vi "Run Test Method.vi"(8 "error in (no error)":errorcluster, 11 "LUnit Test Case In":refnum<class "LUnit Inheriting Test Case.lvclass">) -> (0 "error out":errorcluster, 1 "Execution Time":dbl, 3 "LUnit Test Case Out":refnum<class "LUnit Inheriting Test Case.lvclass">)   [LabVIEW 2020]
uses:
  LUnit Inheriting Test Case.lvclass
  C:/git/astemes-lunit/source/API/LUnit Test Case/LUnit Test Case.lvclass
  C:/git/astemes-lunit/source/Core/Runnable/Runnable.lvclass
  C:/git/astemes-lunit/source/API/LUnit Inheriting Test Case/LUnit Test Case/LUnit Inheriting Test Case.lvclass
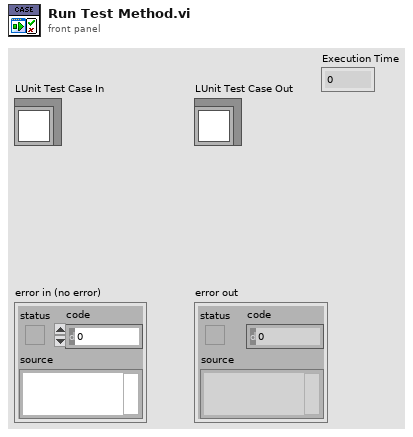
[diagram p1: front panel]
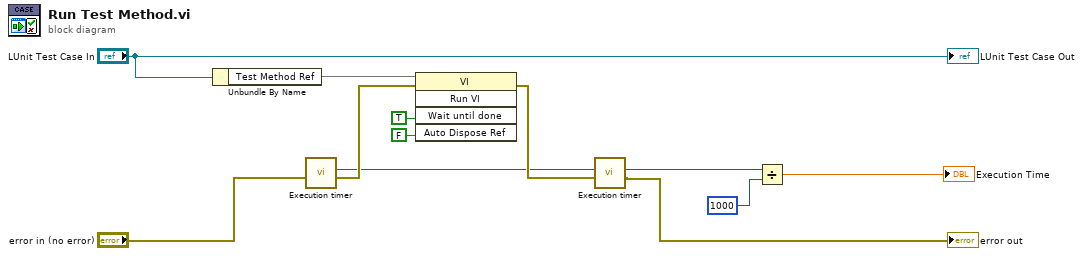
[diagram p0: block diagram]
diagram:
  n1 = Unbundle By Name("LUnit Test Case In") -> ("Test Method Ref"=w8)
  n2 = call "Execution timer.vi"("error in (no error)"="error in (no error)") -> ("error out"=w5:errorcluster, "Current or Duration [ms]"=w3:u32)  [unwired: 9 in]
  n3 = invoke class="VI" method="Run VI"(reference=w8, error in=w5, "Wait until done"=TRUE ("Wait Until Done"), "Auto Dispose Ref"=FALSE ("Auto Dispose Reference")) -> (error out=w4:errorcluster)  [unwired: 1 in, 4 out]
  n4 = call "Execution timer.vi"("error in (no error)"=w4, "millisecond timer value"=w3) -> ("error out"=→"error out":errorcluster, "Current or Duration [ms]"=w2:u32)  [unwired: 8 in]
  n5 = Divide(x=w2, y=u32 1000) -> (x/y=→"Execution Time":dbl)
  "LUnit Test Case Out" <- "LUnit Test Case In"
